vi "dfd_CIC_Decimation.vi"(0 "input data":fxp<+/-,32,32>, 9 "input valid":bool) -> (4 "output data":fxp<+/-,32,32>=-256.0, 10 "output valid":bool=TRUE, 14 "ready for input":bool=TRUE)   [LabVIEW 2017]
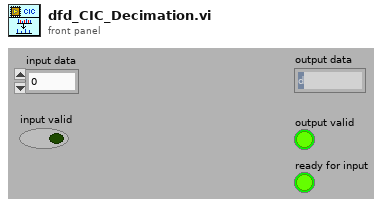
[diagram p1: front panel]
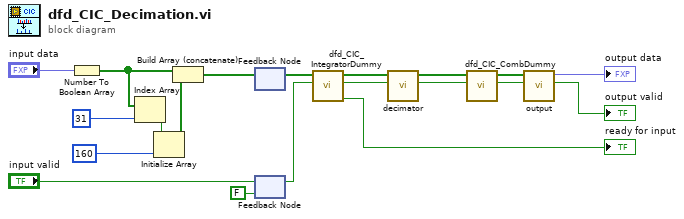
[diagram p0: block diagram]
diagram:
  n1 = Number To Boolean Array(number="input data") -> (Boolean array=w20:bool[])
  n2 = Index Array(array=w20, index=31 ("input msb")) -> (element=w10:bool)
  n3 = Initialize Array(w10, 160 ("192-input wl")) -> (w12:bool[])
  n4 = Build Array (concatenate)(w20, w12) -> (w18:bool[])
  n5 = feedback-in #1(w18) -> ()
  n6 = feedback #1() -> (w3:bool[])  [unwired: 1 out]
  n7 = feedback-in #2("input valid") -> ()
  n8 = feedback #2(FALSE ("input valid")) -> (w2:bool)
  n9 = call <vilib>:"dfd_CIC_IntegratorDummy.vi"("input valid"=w2, "data in"=w3) -> ("ready for input"=→"ready for input":bool, "output valid"=w8:bool, "data out"=w9:bool[])  [unwired: 7 out]
  n10 = call "decimator"("input valid"=w8, "input data"=w9) -> ("output valid"=w6:bool, "output data"=w7:bool[])  [unwired: 8 out]
  n11 = call <vilib>:"dfd_CIC_CombDummy.vi"("input valid"=w6, "data in"=w7) -> ("output valid"=w4:bool, "data out"=w5:bool[])  [unwired: 8 out]
  n12 = call "output"("input valid"=w4, "input data"=w5) -> ("output valid"=→"output valid":bool, "output data"=→"output data":fxp<+/-,32,32>)  [unwired: 8 in]
